vi "String.vi"() -> ()   [LabVIEW 2010]
uses:
  user32.dll
panel:
  in  "String":string
  in  "error in (no error)":errorcluster
  out "error out":errorcluster
  out "Quit":bool
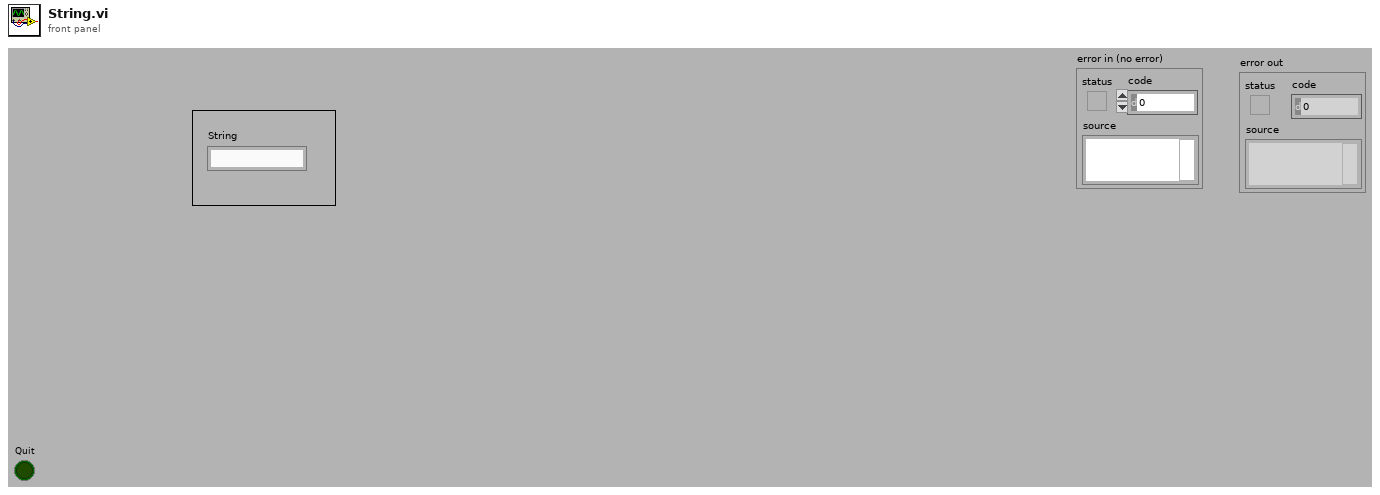
[diagram p1: front panel]
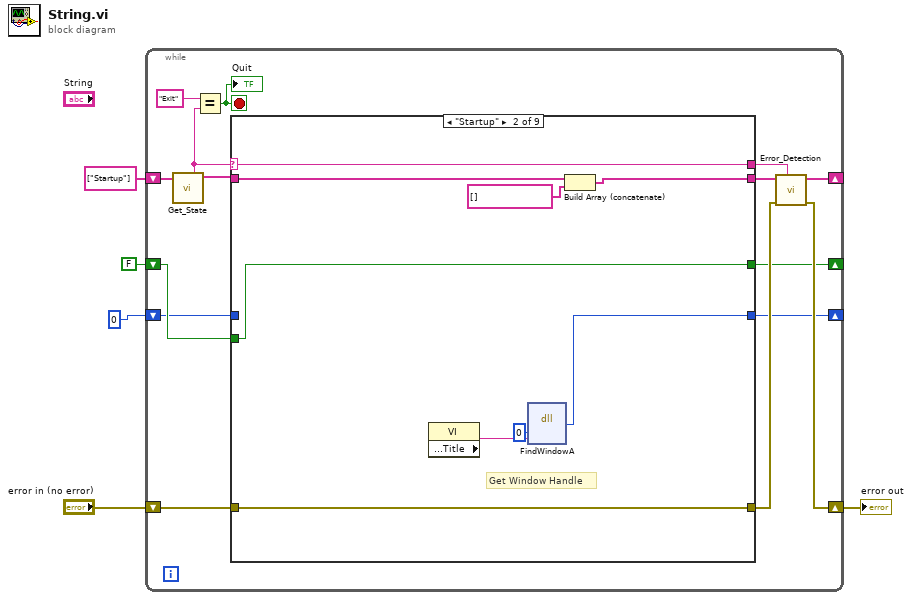
[diagram p0: block diagram]
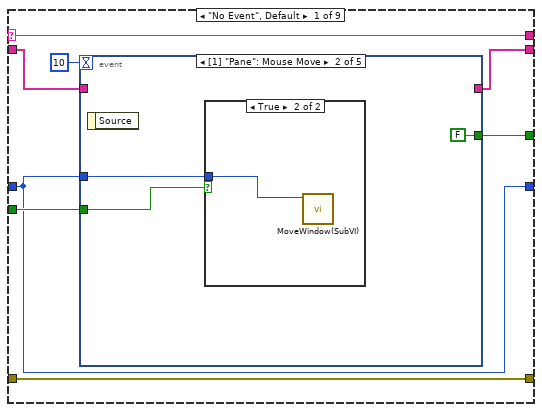
[diagram p2: hidden frame]
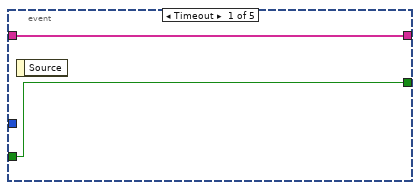
[diagram p3: hidden frame]
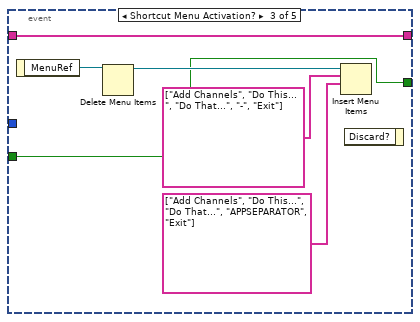
[diagram p5: hidden frame]
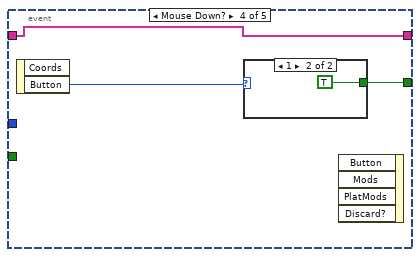
[diagram p6: hidden frame]
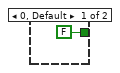
[diagram p7: hidden frame]
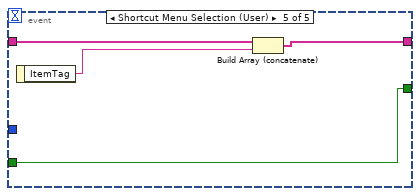
[diagram p8: hidden frame]
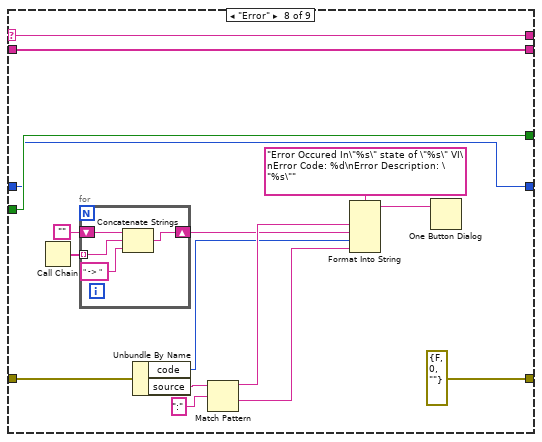
[diagram p14: hidden frame]
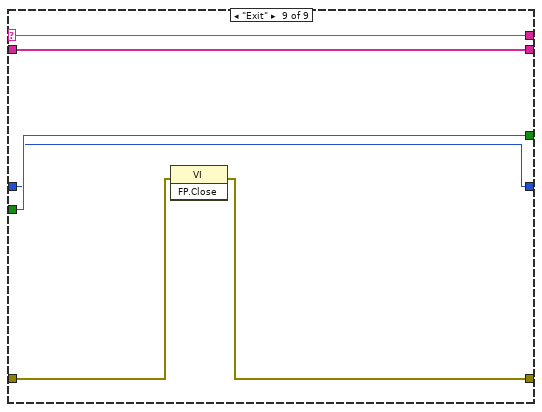
[diagram p15: hidden frame]
diagram:
  n1 = while {
    shift-right: [w13] -> _
    shift-left: string[] ["Startup"] ("State Array Out") -> [w12]
    shift-right: [w14] -> w5
    shift-left: "error in (no error)" -> [w18]
    shift-right: [w9] -> _
    shift-left: FALSE -> [w8]
    shift-right: [w7] -> _
    shift-left: u32 0 ("hWnd") -> [w6]
    stop <- w19 stop-if-true
    n2 = call "Get_State.vi"("State Array In"=w12) -> ("State Array Out"=w11:string[], "Current State"=w10:string)  [unwired: 9 in]
    n3 = Equal?(x="Exit", y=w10) -> (x = y?=w19:bool)
    "Quit" <- w19
    n4 = case shown="\"Startup\"" w10 {
      selector: w10 -> [w28 w58 w62 w67 w72 w77 w83 w99 w109]
      tunnel: w11 -> [w27 w57 w63 w68 w73 w78 w82 w86 w108]
      tunnel: [w24 w56 w63 w68 w73 w78 w82 w86 w108] -> w16
      tunnel: [w25 w54 w61 w66 w71 w76 w81 errorcluster {"status"=FALSE, "code"=0, "source"=""} ("error in (no error)") w105] -> w15
      tunnel: [w28 w58 w62 w67 w72 w77 w83 w99 w109] -> w17
      tunnel: w18 -> [w25 w54 w61 w66 w71 w76 w81 w87 w106]
      tunnel: [w23 w53 w60 w65 w70 w75 w80 w85 w107] -> w9
      tunnel: w8 -> [w22 w53 w60 w65 w70 w75 w80 w85 w107]
      tunnel: [w21 w50 w59 w64 w69 w74 w79 w84 w104] -> w7
      tunnel: w6 -> [w21 _ w59 w64 w69 w74 w79 w84 w104]
      frame "No Event", Default {
        n5 = event shown="[1] \"Pane\": Mouse Move" {
          selector: _ -> [_ _ _ _ _]
          dyn-events: _ -> [_ _ _ _ _]
          timeout: 10 -> [_ _ _ _ _]
          tunnel: [w30 _ w38 w43 w48] -> w24
          tunnel: w27 -> [w30 _ w38 w43 w49]
          tunnel: [w29 FALSE w35 w42 w46] -> w23
          tunnel: w22 -> [w29 w33 w35 _ w46]
          tunnel: w21 -> [_ w31 _ _ _]
          event Timeout {
            n6 = event-data() -> ()  [unwired: 1 in, 1 out]
          }
          event Mouse Move {
            n7 = event-data() -> ()  [unwired: 1 in, 1 out]
            n8 = case shown="True" w33 {
              tunnel: w31 -> [_ w34]
              frame False {
              }
              frame True {
                n9 = call "MoveWindow(SubVI).vi"("hWnd"=w34) -> ()  [unwired: 10 in, 1 out]
              }
            }
          }
          event Shortcut Menu Activation? {
            n10 = event-data() -> ("MenuRef"=w37:refnum<k9>)  [unwired: 1 in]
            n11 = Delete Menu Items(9:w37) -> (3:w36:refnum<k9>)  [unwired: 3 in, 1 out]
            n12 = Insert Menu Items(7:string[] ["Add Channels", "Do This...", "Do That...", "APPSEPARATOR", "Exit"], 8:string[] ["Add Channels", "Do This...", "Do That...", "-", "Exit"], 9:w36) -> ()  [unwired: 3 in, 3 out]
            n13 = event-data() -> ()  [unwired: 2 in, 1 out]
          }
          event Mouse Down? {
            n14 = event-data() -> ("Button"=w41:u16)  [unwired: 1 in, 1 out]
            n15 = case shown="1" w41 {
              tunnel: [FALSE TRUE] -> w42
              frame 0, Default {
              }
              frame 1 {
              }
            }
            n16 = event-data() -> ()  [unwired: 5 in, 1 out]
          }
          event Shortcut Menu Selection (User) {
            n17 = event-data() -> ("ItemTag"=w47:string)  [unwired: 1 in]
            n18 = Build Array (concatenate)(w49, w47) -> (w48:string[])
          }
        }
      }
      frame "Startup" {
        # "Get Window Handle"
        n19 = property class="VI"() -> ("Front Panel.Title"=w51:string)  [unwired: 2 in, 2 out]
        n20 = dll-call lib="user32.dll" fn="FindWindowA"("arg1"=0, "arg2"=w51) -> ("return type"=w50:i32)  [unwired: 5 in, 2 out]
        n21 = Build Array (concatenate)(w57, string[] [] ("State Array Out")) -> (w56:string[])
      }
      frame "---------------UI Events---------------" {
        # "This State will never Execute\nIt is added just for improving code readability.\nPlease do not remove."
      }
      frame "---------------Menu Events---------------" {
        # "This State will never Execute\nIt is added just for improving code readability.\nPlease do not remove."
      }
      frame "---------------Client Events---------------" {
        # "This State will never Execute\nIt is added just for improving code readability.\nPlease do not remove."
      }
      frame "---------------Subroutine states---------------" {
        # "This State will never Execute\nIt is added just for improving code readability.\nPlease do not remove."
      }
      frame "---------------Error Handling VIs---------------" {
        # "This State will never Execute\nIt is added just for improving code readability.\nPlease do not remove."
      }
      frame "Error" {
        n22 = Call Chain() -> (call chain=w94:string[])
        n23 = for {
          tunnel: w94 -> [w102] mode=indexing
          shift-right: [w100] -> w91
          shift-left: "" -> [w103]
          n24 = Concatenate Strings(w103, w102, " -> ") -> (w100:string)
        }
        n25 = Unbundle By Name(w87) -> ("code"=w89:i32, "source"=w88:string)
        n26 = Match Pattern(string=w88, regular expression=":") -> (before substring=w92:string, after substring=w96:string)  [unwired: 1 in, 2 out]
        n27 = Format Into String(format string="Error Occured In\"%s\" state of \"%s\" VI\nError Code: %d\nError Description: \"%s\"", w92, w91, w89, w96) -> (resulting string=w95:string)  [unwired: 2 in, 1 out]
        n28 = One Button Dialog(message=w95) -> ()  [unwired: 1 in, 1 out]
      }
      frame "Exit" {
        n29 = invoke class="VI" method="FP.Close"(error in=w106) -> (error out=w105:errorcluster)  [unwired: 2 in, 2 out]
      }
    }
    n30 = call "Error_Detection.vi"("Current State"=w17, "error in (no error)"=w15, "Msg In"=w16) -> ("error out"=w14:errorcluster, "Msg Out"=w13:string[])  [unwired: 7 in]
  }
  "error out" <- w5
